vi "My Nonlinear Curve Fit TR bounds.vi"(0 "Y":dbl[](array[numeric]), 1 "f(x,a)":T5, 2 "data":variant, 5 "X":dbl[](array[numeric]), 7 "Weight":dbl[](array[numeric]), 9 "initial parameters":dbl[](array[numeric]), 11 "error in (no error)":errorcluster, 12 "Termination Criteria":T6={"Max Iterations"=1000, "Max Function Calls"=10000, "Max Time"=1000.0, "Function Tolerance"=1e-06, "Parameter Tolerance"=1e-06, "Gradient Tolerance"=1e-06, "Min Lambda"=1e-06, "Max Lambda"=1000000.0, "Initial Tick Count"=0}, 13 "parameter bounds":T3, 14 "method":T4 items=["Least Square", "Least Absolute Residual", "Bisquare"]) -> (3 "Fit Aborted?":bool, 4 "best nonlinear fit":dbl[](array[numeric]), 6 "best fit parameters":dbl[](array[numeric]), 8 "covariance":T7, 10 "Fit Statistics":T1={"# Iterations"=0, "# Function Calls"=0, "Chi2"=0.0, "Chi2/DOF"=0.0, "Fit Convergence Criterion"=enum."Continue", "Gradient"=0.0, "|Delta Chi 2|"=0.0, "|Delta Chi 2|/Chi 2"=0.0, "Max |Delta a| /|a|"=0.0, "Lambda"=-1.0}, 15 "error out":errorcluster)   [LabVIEW 2021, in "Fits.lvlib"]
uses:
  Fits.lvlib
  <vilib>/Analysis/Matrix/Datatypes/RealMatrix.ctl
  My Fit Stopping Criteria.ctl
  <vilib>/gmath/NumericalOptimization/LM model function reference.ctl
  <vilib>/Analysis/6fits.llb/Curve Fitting Criteria.ctl
  Fit Statistics v2.ctl
  Convergence Criteria.ctl
  <vilib>/gmath/NumericalOptimization/LM model function.ctl
  <vilib>/gmath/NumericalOptimization/LM_output select.ctl
  Abort Fit Global.vi
  <vilib>/Analysis/baseanly.llb/Real Inverse Matrix.vi
  <vilib>/gmath/NI_Gmath.lvlib
  <vilib>/Analysis/NI_AALBase.lvlib
  <vilib>/Analysis/Matrix/NI_Matrix.lvlib
  <vilib>/Analysis/NI_AALPro.lvlib
panel:
  in  "TR update constants":cluster{"h1":dbl, "h2":dbl, "a1":dbl, "a2":dbl}={"h1"=0.0001, "h2"=0.99, "a1"=0.25, "a2"=3.5}
  out "TR Radius Chart":dbl(graph)
  out "Parameters Gradient Chart":dbl[][](graph)
  in  "Repeat Fit N times (1)":i32=1
  in  "Reset Charts":bool
  out "Chi2 Chart":dbl(graph)
  out "Parameters Graph":dbl[](graph)
  in  "Delay (ms)":i32
  in  "Debug":bool
  out "Parameters Chart":dbl[][](graph)
  out "Function & Fit Graph":cluster{"New Coefficients":dbl[]}[](graph)
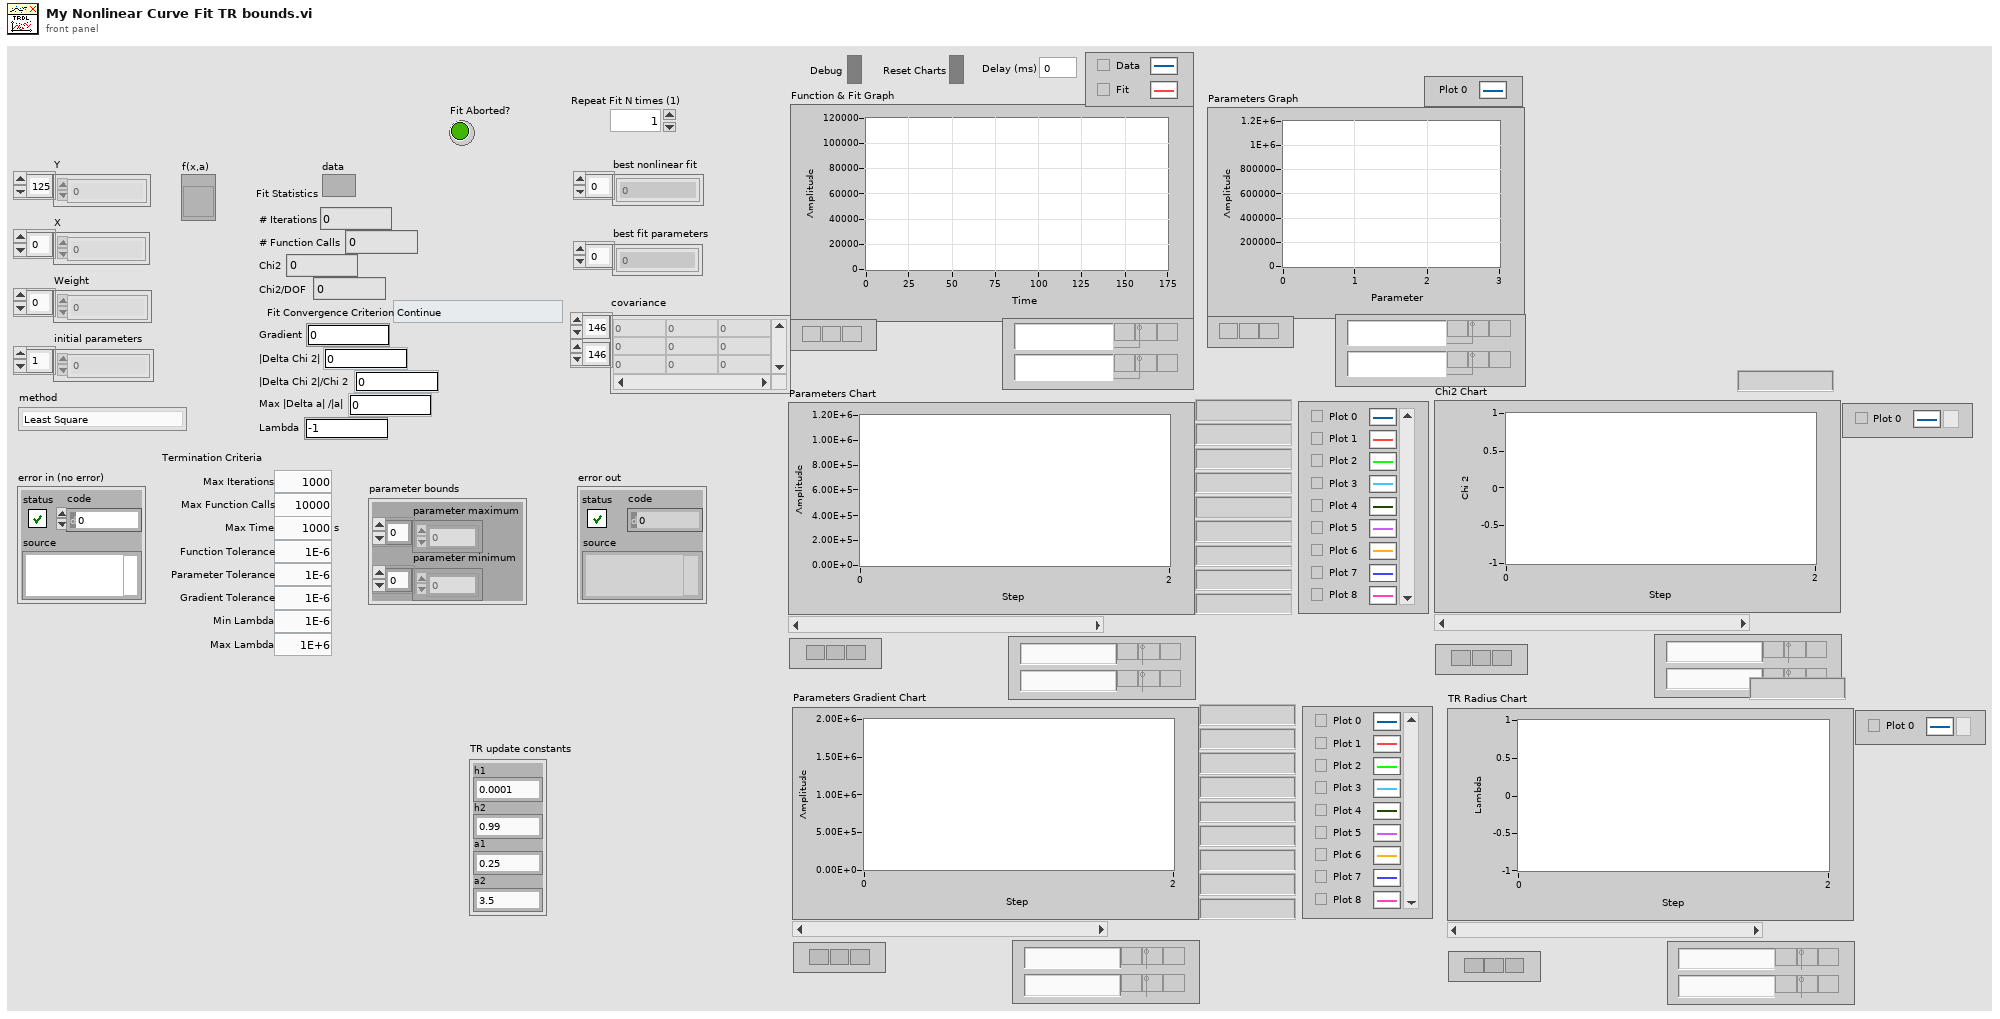
[diagram p1: front panel]
types:
  T1 = typedef "Fits.lvlib/Fit Statistics v2.ctl" = cluster{"# Iterations":i32, "# Function Calls":i32, "Chi2":dbl, "Chi2/DOF":dbl, "Fit Convergence Criterion":T2, "Gradient":dbl, "|Delta Chi 2|":dbl, "|Delta Chi 2|/Chi 2":dbl, "Max |Delta a| /|a|":dbl, "Lambda":dbl}
  T2 = typedef "Fits.lvlib/Convergence Criteria.ctl" = enum16{"Continue", "Tolerances Exceeded", "Max Time Exceeded", "Max Iterations Exceeded", "Max Function Evaluations Exceeded", "Scale Range Exceeded"}
  T3 = cluster{"parameter minimum":dbl[], "parameter maximum":dbl[]}
  T4 = typedef "NI_AALPro.lvlib/Curve Fitting Criteria.ctl" = u16
  T5 = typedef "NI_Gmath.lvlib/LM model function reference.ctl" = refnum<vi>
  T6 = typedef "Fits.lvlib/My Fit Stopping Criteria.ctl" = cluster{"Max Iterations":i32, "Max Function Calls":i32, "Max Time":dbl[unit], "Function Tolerance":dbl, "Parameter Tolerance":dbl, "Gradient Tolerance":dbl, "Min Lambda":dbl, "Max Lambda":dbl, "Initial Tick Count":u32}
  T7 = typedef "NI_Matrix.lvlib/RealMatrix.ctl" = dbl[][]
  T8 = typedef "NI_Gmath.lvlib/LM model function.ctl" = cluster{"f(x,a)":T5, "data":variant}
  T9 = typedef "NI_Gmath.lvlib/LM_output select.ctl" = cluster{"model function":bool, "gradient":bool}
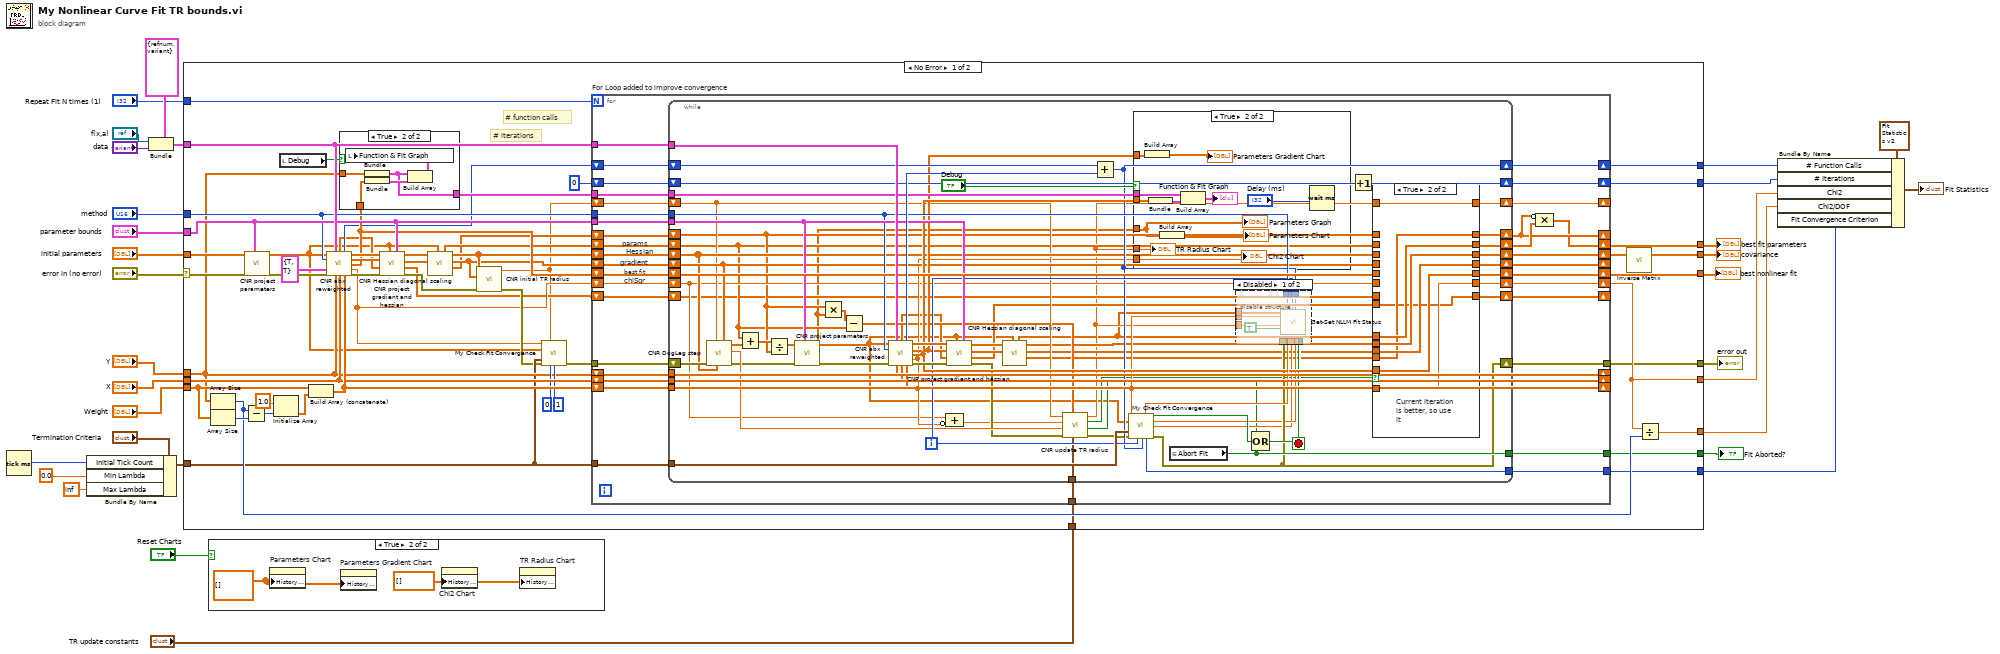
[diagram p0: block diagram]
diagram:
  n1 = Tick Count (ms)() -> (millisecond timer value=w9:u32)
  n2 = Bundle By Name(cluster="Termination Criteria", "Initial Tick Count"=w9, "Min Lambda"=0.0, "Max Lambda"=inf) -> (w8:T6)
  n3 = Bundle(cluster=T8 {"f(x,a)"=refnum, "data"=variant} ("model function"), "f(x,a)"="f(x,a)", "data"="data") -> (w20:T8)
  n4 = case shown="No Error" "error in (no error)" {
    selector: "error in (no error)" -> [w64 w233]
    tunnel: [w67 _] -> w31
    tunnel: [w84 _] -> w11
    tunnel: "initial parameters" -> [w65 _]
    tunnel: [w74 _] -> w29
    tunnel: [w82 _] -> w28
    tunnel: "Weight" -> [w78 _]
    tunnel: "Y" -> [w56 _]
    tunnel: w8 -> [w49 _]
    tunnel: "X" -> [w75 _]
    tunnel: [w48 w233] -> w24
    tunnel: w20 -> [w76 _]
    tunnel: [w69 _] -> w15
    tunnel: "method" -> [w58 _]
    tunnel: "parameter bounds" -> [w59 _]
    tunnel: [w57 _] -> w16
    tunnel: [w52 _] -> w12
    tunnel: [w50 _] -> w13
    tunnel: "Repeat Fit N times (1)" -> [w47 _]
    tunnel: [w46 _] -> w4
    tunnel: "TR update constants" -> [w36 _]
    frame No Error {
      # "# function calls"
      # "# iterations"
      n5 = Array Size(array=w56) -> (size(s)=w66:i32)
      n6 = Array Size(array=w78) -> (size(s)=w81:i32)
      n7 = Subtract(x=w66, y=w81) -> (x-y=w80:i32)
      n8 = call <vilib>:"CNR project parameters.vi"("bounds"=w59, "error in"=w64, "parameters"=w65) -> ("error out"=w63:errorcluster, "projected parameters"=w33:dbl[])  [unwired: 7 out]
      n9 = Initialize Array(1.0, w80) -> (w79:dbl[])
      n10 = local read "Debug"() -> (w53:bool)
      n11 = Build Array (concatenate)(w78, w79) -> (w85:dbl[])
      n12 = call <vilib>:"CNR abx reweighted.vi"("parameters"=w33, "model function"=w76, "method"=w58, "output control"=T9 {"model function"=TRUE, "gradient"=TRUE}, "error in (no error)"=w63, "Y"=w56, "X"=w75, "Weight"=w85) -> ("Jacobian"=w34:T7, "number of function calls"=w51:i32, "Hessian"=w61:T7, "gradient"=w60:dbl[], "best fit"=w54:dbl[], "chiSqr"=w37:dbl, "error out"=w62:errorcluster)  [unwired: 1 in]
      n13 = case shown="True" w53 {
        tunnel: w56 -> [_ w232]
        tunnel: [_ w229] -> w55
        tunnel: w54 -> [_ w231]
        frame False {
        }
        frame True {
          n14 = Bundle("Y"=w232) -> (w229:cluster{"Y":dbl[]})  [unwired: 1 in]
          n15 = Bundle("best fit"=w231) -> (w230:cluster{"best fit":dbl[]})  [unwired: 1 in]
          n16 = Build Array(w229, w230) -> (w228:cluster{"best fit":dbl[]}[])
          n17 = local write "Function & Fit Graph"(w228) -> ()
        }
      }
      n18 = call <vilib>:"CNR project gradient and hessian.vi"("bounds"=w59, "projected parameters"=w33, "error in"=w62, "Jacobian"=w34, "gradient"=w60, "Hessian"=w61) -> ("error out"=w40:errorcluster, "projected jacobian"=w35:T7, "projected gradient"=w44:dbl[], "projected Hessian"=w45:T7)  [unwired: 2 out]
      n19 = call <vilib>:"CNR Hessian diagonal scaling.vi"("parameters"=w33, "gradient"=w44, "Hessian"=w45) -> ("D"=w38:dbl[], "scaled gradient"=w41:dbl[], "scaled Hessian"=w43:T7, "scaled parameters"=w42:dbl[])  [unwired: 5 out]
      n20 = call <vilib>:"CNR initial TR radius.vi"("error in"=w40, "g"=w41, "H"=w43) -> ("error out"=w39:errorcluster, "initial TR radius"=w32:dbl)  [unwired: 7 out]
      n21 = call "My Check Fit Convergence.vi"("Chi 2"=w37, "Lambda"=w32, "Parameters"=w33, "my stopping criteria"=w49, "Error In"=w39, "current iteration"=0, "number of function evaluations"=1) -> ("error out"=w77:errorcluster)  [unwired: 1 in, 7 out]
      n22 = for "For Loop added to improve convergence" {
        N: w47 -> [_]
        tunnel: w76 -> [w117]
        tunnel: w59 -> [w111]
        tunnel: w58 -> [w108]
        tunnel: [w107] -> w57
        tunnel: w55 -> [w106]
        tunnel: w49 -> [w101]
        shift-right: [w104] -> w52
        shift-left: w37 -> [w119]
        shift-right: [w113] -> w69
        shift-left: w51 -> [w103]
        shift-right: [w102] -> w50
        shift-left: 0 -> [w114]
        shift-right: [w86] -> w67
        shift-left: w42 -> [w112]
        shift-right: [w115] -> w71
        shift-left: w43 -> [w110]
        shift-right: [w99] -> _
        shift-left: w41 -> [w109]
        shift-right: [w116] -> w74
        shift-left: w54 -> [w105]
        shift-right: [w98] -> _
        shift-left: w56 -> [w98]
        shift-right: [w97] -> _
        shift-left: w75 -> [w97]
        shift-right: [w96] -> _
        shift-left: w85 -> [w96]
        tunnel: [w94] -> w46
        tunnel: w77 -> [w118]
        tunnel: [w95] -> w48
        shift-right: [w87] -> _
        shift-left: w38 -> [w93]
        shift-right: [w92] -> _
        shift-left: w32 -> [w100]
        tunnel: w36 -> [w91]
        shift-right: [w90] -> _
        shift-left: w35 -> [w89]
        # "best fit"
        # "chiSqr"
        # "gradient"
        # "Hessian"
        # "params"
        n23 = while {
          tunnel: w97 -> [w184]
          tunnel: w98 -> [w167]
          tunnel: w96 -> [w183]
          shift-left: w119 -> [w140]
          shift-right: [w175] -> w104
          shift-left: w109 -> [w152]
          shift-right: [w186] -> w99
          shift-left: w110 -> [w151]
          shift-right: [w187] -> w115
          shift-left: w112 -> [w135]
          shift-right: [w176] -> w88
          shift-left: w100 -> [w144]
          shift-right: [w185] -> w92
          shift-right: [w158] -> w95
          shift-left: w118 -> [w153]
          tunnel: w117 -> [w182]
          tunnel: w101 -> [w178]
          shift-right: [w160] -> w113
          shift-left: w103 -> [w181]
          shift-right: [w179] -> w116
          shift-left: w105 -> [w180]
          shift-right: [w162] -> w102
          shift-left: w114 -> [w163]
          tunnel: w108 -> [w169]
          tunnel: w111 -> [w172]
          tunnel: [w170] -> w107
          tunnel: w106 -> [w166]
          tunnel: [w155] -> w94
          shift-right: [w137] -> w87
          shift-left: w93 -> [w138]
          tunnel: w91 -> [w143]
          shift-right: [w128] -> w90
          shift-left: w89 -> [w127]
          i -> [w161]
          stop <- w159 stop-if-true
          n24 = call <vilib>:"CNR DogLeg step.vi"("gradient"=w152, "Hessian"=w151, "TR radius"=w144, "error in (no error)"=w153) -> ("error out"=w142:errorcluster, "L(0)-L(hdl)\npredicted change"=w149:dbl, "x step"=w150:dbl[])  [unwired: 3 in, 2 out]
          n25 = Add(x=w135, y=w150) -> (x+y=w146:dbl[])
          n26 = Divide(x=w146, y=w138) -> (x/y=w145:dbl[])
          n27 = call <vilib>:"CNR project parameters.vi"("bounds"=w172, "error in"=w142, "parameters"=w145) -> ("error out"=w174:errorcluster, "projected parameters"=w120:dbl[])  [unwired: 7 out]
          n28 = Multiply(x=w138, y=w120) -> (x*y=w136:dbl[])
          n29 = Subtract(x=w136, y=w135) -> (x-y=w134:dbl[])
          n30 = call <vilib>:"CNR abx reweighted.vi"("parameters"=w120, "model function"=w182, "method"=w169, "error in (no error)"=w174, "Y"=w167, "X"=w184, "Weight"=w183) -> ("Jacobian"=w130:T7, "number of function calls"=w188:i32, "Hessian"=w171:T7, "gradient"=w154:dbl[], "best fit"=w164:dbl[], "chiSqr"=w141:dbl, "error out"=w173:errorcluster)  [unwired: 2 in]
          n31 = Compound Arithmetic op=ADD(w140, invert w141) -> (w139:dbl)
          n32 = call <vilib>:"CNR project gradient and hessian.vi"("bounds"=w172, "projected parameters"=w120, "error in"=w173, "Jacobian"=w130, "gradient"=w154, "Hessian"=w171) -> ("error out"=w148:errorcluster, "projected jacobian"=w129:T7, "projected gradient"=w131:dbl[], "projected Hessian"=w133:T7)  [unwired: 2 out]
          n33 = call <vilib>:"CNR Hessian diagonal scaling.vi"("parameters"=w120, "gradient"=w131, "Hessian"=w133) -> ("D"=w126:dbl[], "scaled gradient"=w123:dbl[], "scaled Hessian"=w132:T7, "scaled parameters"=w121:dbl[])  [unwired: 5 out]
          n34 = call <vilib>:"CNR update TR radius.vi"("TR update constants"=w143, "step"=w134, "error in (no error)"=w148, "L(0)-L(p_dl)"=w149, "F(x)-F(x+p)"=w139, "TR Radius"=w144) -> ("error out"=w147:errorcluster, "quit?"=w124:bool, "step OK?"=w125:bool, "TR Radius out"=w122:dbl)  [unwired: 2 out]
          n35 = Add(x=w181, y=w188) -> (x+y=w160:i32)
          n36 = call "My Check Fit Convergence.vi"("Chi 2"=w141, "Parameters"=w120, "my stopping criteria"=w178, "Error In"=w147, "current iteration"=w161, "number of function evaluations"=w160) -> ("|Delta Chi 2|/Chi 2"=w168:dbl, "stop?"=w177:bool, "|Delta Chi 2|"=w157:dbl, "Max |Delta a| /|a|"=w156:dbl, "Convergence Criterium Reached"=w155:T2, "error out"=w158:errorcluster)  [unwired: 2 in, 2 out]
          n37 = case shown="True" "Debug" {
            tunnel: w120 -> [_ w204]
            tunnel: w166 -> [_ w211]
            tunnel: w164 -> [_ w208]
            tunnel: w141 -> [_ w206]
            tunnel: w154 -> [_ w205]
            tunnel: w122 -> [_ w201]
            frame False {
            }
            frame True {
              n38 = Build Array(w205) -> (→"Parameters Gradient Chart":dbl[][])
              n39 = Bundle("best fit"=w208) -> (w210:cluster{"best fit":dbl[]})  [unwired: 1 in]
              n40 = Build Array(w204) -> (→"Parameters Chart":dbl[][])
              n41 = Build Array(w211, w210) -> (→"Function & Fit Graph":cluster{"best fit":dbl[]}[])
              n42 = Wait (ms)(milliseconds to wait="Delay (ms)") -> ()  [unwired: 1 out]
              "Parameters Graph" <- w204
              "Chi2 Chart" <- w206
              "TR Radius Chart" <- w201
            }
          }
          n43 = global read "Abort Fit Global.vi" "Abort Fit"() -> (w170:bool)
          n44 = Compound Arithmetic op=OR(w124, w177, w170) -> (w159:bool)
          n45 = disable-structure shown="Disabled" {
            disable-tunnel: w169 -> [w200 _]
            disable-tunnel: w168 -> [w198 _]
            disable-tunnel: w161 -> [w197 _]
            disable-tunnel: w160 -> [w196 _]
            disable-tunnel: w159 -> [w195 _]
            disable-tunnel: w158 -> [w194 _]
            disable-tunnel: w157 -> [w193 _]
            disable-tunnel: w156 -> [w192 _]
            disable-tunnel: w141 -> [w191 _]
            disable-tunnel: w122 -> [w190 _]
            disable-tunnel: w121 -> [w189 _]
            frame Disabled {
              n46 = call "Get-Set NLLM Fit Status.vi"("Fit Parameters"=w189, "chiSqr"=w191, "Lambda"=w190, "Get(F)/Set"=TRUE, "Error In"=w194, "NL Fit Method"=w200, "|Delta Chi 2|/Chi 2"=w198, "# Iterations"=w197, "Max |Delta a| /|a|"=w192, "# Function Calls"=w196, "|Delta Chi 2|"=w193, "Done"=w195) -> ()  [unwired: 6 in, 2 out]
            }
            frame Enabled {
            }
          }
          n47 = Increment(x=w163) -> (x+1=w162:i32)
          n48 = case shown="True" w125 {
            tunnel: [w219 w227] -> w187
            tunnel: w151 -> [w219 _]
            tunnel: [w218 w226] -> w186
            tunnel: w121 -> [_ w223]
            tunnel: w152 -> [w218 _]
            tunnel: w135 -> [w217 _]
            tunnel: [w217 w223] -> w176
            tunnel: [w214 w222] -> w185
            tunnel: w140 -> [w216 _]
            tunnel: w141 -> [_ w224]
            tunnel: [w216 w224] -> w175
            tunnel: w122 -> [w214 w222]
            tunnel: w132 -> [_ w227]
            tunnel: w123 -> [_ w226]
            tunnel: w180 -> [w215 _]
            tunnel: w164 -> [_ w225]
            tunnel: [w215 w225] -> w179
            tunnel: w138 -> [w213 _]
            tunnel: [w213 w221] -> w137
            tunnel: w126 -> [_ w221]
            tunnel: w129 -> [_ w220]
            tunnel: [w212 w220] -> w128
            tunnel: w127 -> [w212 _]
            frame False {
              # "Previous iteration\nis better, so keep\nit"
            }
            frame True {
              # "Current iteration\nis better, so use\nit"
            }
          }
        }
        n49 = Compound Arithmetic op=MULTIPLY(invert w87, w88) -> (w86:dbl[])
      }
      n50 = call-poly <vilib>:"Inverse Matrix.vi"("Input Matrix"=w71) -> ("Inverse Matrix"=w82:T7)  [unwired: 1 in, 1 out]
      n51 = Divide(x=w52, y=w66) -> (x/y=w84:dbl)
    }
    frame Error {
    }
  }
  "best fit parameters" <- w31
  "best nonlinear fit" <- w29
  "error out" <- w24
  "covariance" <- w28
  "Fit Aborted?" <- w16
  n52 = case shown="True" "Reset Charts" {
    frame False {
    }
    frame True {
      w234 = dbl[] [] ("History Data")
      w235 = dbl[][] [] ("History Data")
      n53 = property on="Parameters Chart" class="WFChart (strict)"("History Data"=w235) -> ()  [unwired: 2 in, 2 out]
      n54 = property on="Parameters Gradient Chart" class="WFChart (strict)"("History Data"=w235) -> ()  [unwired: 2 in, 2 out]
      n55 = property on="Chi2 Chart" class="WFChart (strict)"("History Data"=w234) -> ()  [unwired: 2 in, 2 out]
      n56 = property on="TR Radius Chart" class="WFChart (strict)"("History Data"=w234) -> ()  [unwired: 2 in, 2 out]
    }
  }
  n57 = Bundle By Name(cluster=T1 {"# Iterations"=0, "# Function Calls"=0, "Chi2"=0.0, "Chi2/DOF"=0.0, "Fit Convergence Criterion"=enum."Continue", "Gradient"=0.0, "|Delta Chi 2|"=0.0, "|Delta Chi 2|/Chi 2"=0.0, "Max |Delta a| /|a|"=0.0, "Lambda"=-1.0} ("Fit Statistics"), "# Function Calls"=w15, "# Iterations"=w13, "Chi2"=w12, "Chi2/DOF"=w11, "Fit Convergence Criterion"=w4) -> (→"Fit Statistics":T1)
